vi "FG In Obstacle Field.vi"(2 "FG Action (Read)":T1, 3 "In Obs. Field? in":bool) -> (1 "In Obs. Field? out":bool)   [LabVIEW 2009]
uses:
  Actions for FG's.ctl
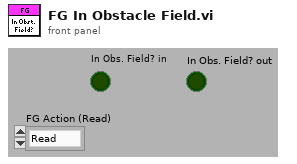
[diagram p1: front panel]
types:
  T1 = typedef "Actions for FG's.ctl" = enum16{"Read", "Write"}
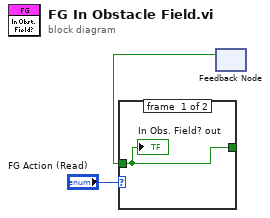
[diagram p0: block diagram]
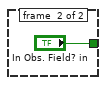
[diagram p2: hidden frame]
diagram:
  n1 = feedback #1() -> (w1:bool)  [unwired: 1 in]
  n2 = case shown="\"Write\"" "FG Action (Read)" {
    tunnel: [w4 "In Obs. Field? in"] -> w2
    tunnel: w1 -> [w4 _]
    frame #0 {
      "In Obs. Field? out" <- w4
    }
    frame #1 {
    }
  }
